vi "Check Can Write.vi"(8 "error in (no error)":errorcluster, 11 "Config Manager in":refnum<class "Config Manager.lvclass">) -> (0 "error out":errorcluster, 3 "Config Manager out":refnum<class "Config Manager.lvclass">)   [LabVIEW 2023, in "CDM-Config.lvlib" / "Config Manager.lvclass"]
uses:
  Config Manager.lvclass
  Config Manager.lvclass/Config Manager.ctl
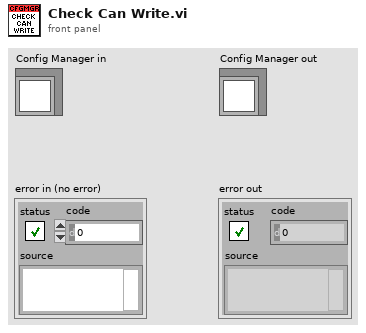
[diagram p1: front panel]
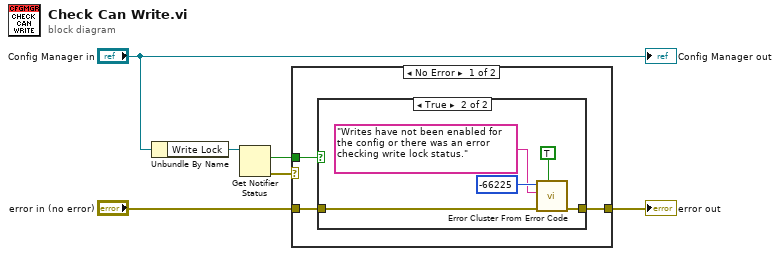
[diagram p0: block diagram]
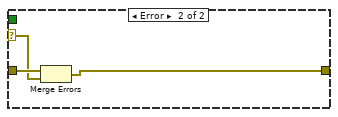
[diagram p3: hidden frame]
diagram:
  n1 = Unbundle By Name("Config Manager in") -> ("Write Lock"=w6:refnum<notifier>)
  n2 = Get Notifier Status(notifier=w6) -> (current notification=w2:bool, error out=w1:errorcluster)  [unwired: 1 in, 3 out]
  n3 = case shown="No Error" w1 {
    selector: w1 -> [_ w17]
    tunnel: "error in (no error)" -> [w9 w18]
    tunnel: [w8 w16] -> w3
    tunnel: w2 -> [w7 _]
    frame No Error {
      n4 = case shown="True" w7 {
        tunnel: w9 -> [w10 w15]
        tunnel: [w10 w14] -> w8
        frame False {
        }
        frame True {
          n5 = call <vilib>:"Error Cluster From Error Code.vi"("show call chain? (False)"=TRUE, "error in (no error)"=w15, "error message (\"\")"="Writes have not been enabled for the config or there was an error checking write lock status.", "error code (0)"=-66225) -> ("error out"=w14:errorcluster)  [unwired: 5 in]
        }
      }
    }
    frame Error {
      n6 = Merge Errors(w18, w17) -> (w16:errorcluster)
    }
  }
  "error out" <- w3
  "Config Manager out" <- "Config Manager in"
